vi "FGV-B-Scan Active.vi"(7 "Action":T1 caption="Action (def: Read)", 8 "error in (no error)":errorcluster) -> (0 "error out":errorcluster, 1 "B-Scan In Progress?":bool, 2 "B-Scan Start?":bool)   [LabVIEW 2026, in "MicroPulse_Driver.lvlib"]
uses:
  MicroPulse_Driver.lvlib
  Low Level/FGV - B-Scan Active - Action [Enum].ctl
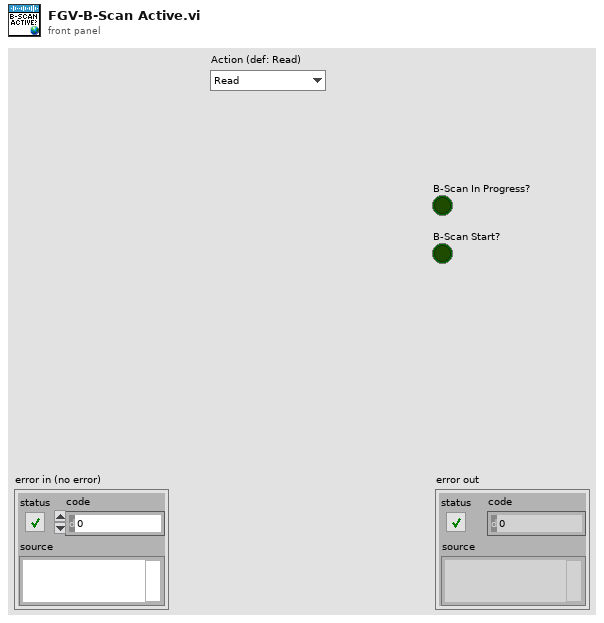
[diagram p1: front panel]
types:
  T1 = typedef "MicroPulse_Driver.lvlib/FGV - B-Scan Active - Action [Enum].ctl" = enum16{"Read", "Read & Reset Start Flag", "Start B-Scan", "B-Scan Finished"}
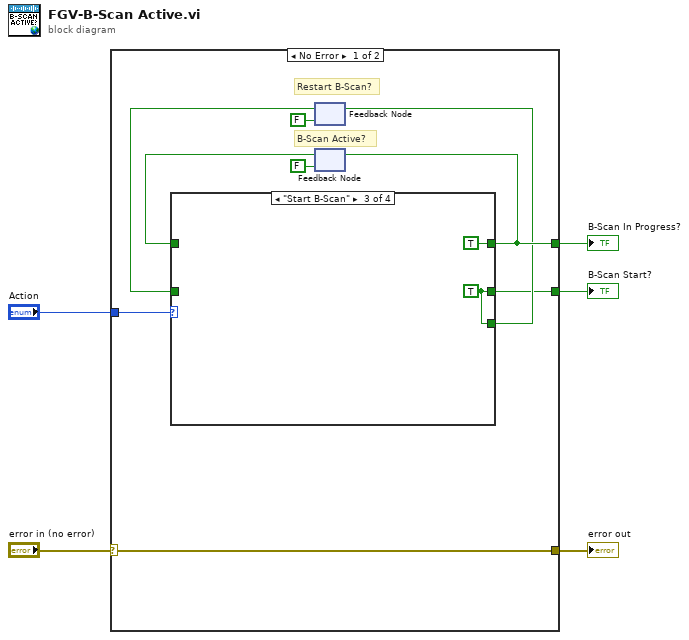
[diagram p0: block diagram]
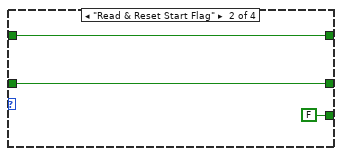
[diagram p3: hidden frame]
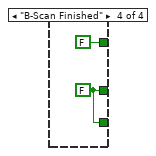
[diagram p4: hidden frame]
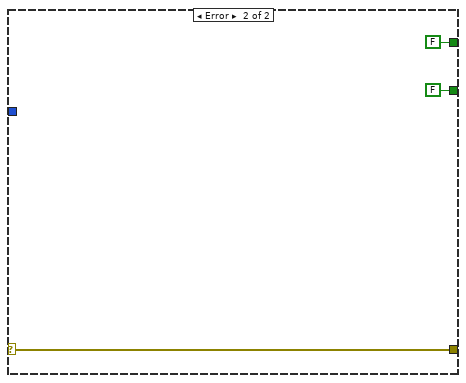
[diagram p5: hidden frame]
diagram:
  n1 = case shown="No Error" "error in (no error)" {
    selector: "error in (no error)" -> [w14 w26]
    tunnel: [w14 w26] -> w4
    tunnel: "Action" -> [w13 _]
    tunnel: [w10 FALSE] -> w2
    tunnel: [w6 FALSE] -> w1
    frame No Error {
      # "B-Scan Active?"
      # "Restart B-Scan?"
      n2 = feedback #1(FALSE) -> (w8:bool)
      n3 = feedback #2(FALSE) -> (w11:bool)
      n4 = case shown="\"Start B-Scan\"" w13 {
        tunnel: [w16 w19 TRUE FALSE] -> w10
        tunnel: w11 -> [w16 w19 _ _]
        tunnel: [w15 FALSE w20 w22] -> w7
        tunnel: w8 -> [w15 w17 _ _]
        tunnel: [w15 w17 w20 w22] -> w6
        frame "Read", Default {
        }
        frame "Read & Reset Start Flag" {
        }
        frame "Start B-Scan" {
          w20 = TRUE
        }
        frame "B-Scan Finished" {
          w22 = FALSE
        }
      }
      n5 = feedback-in #1(w7) -> ()
      n6 = feedback-in #2(w10) -> ()
    }
    frame Error {
    }
  }
  "error out" <- w4
  "B-Scan In Progress?" <- w2
  "B-Scan Start?" <- w1
